vi "CRYMake Play and Record Array.vi"(0 "Play&Record/Record":bool, 1 "Name Mode":bool, 2 "Selected Record Signal Path In":string[](array[string]), 3 "Selected Play Signal Path In":string[](array[string]), 5 "Selected Record In":string[][](array[string]), 7 "input channel Info In":T5[](array[typedef]) {"Coupling" items=["Default"=-1, "RSE"=10083, "NRSE"=10078, "Differential"=10106, "Pseudodifferential"=12529]; "term config" items=["Default"=-1, "RSE"=10083, "NRSE"=10078, "Differential"=10106, "Pseudodifferential"=12529]; "Anti-aliasing Factor (%fs)" format="%.2f"}, 9 "Selected Play In":string[][](array[string]), 11 "output channel Info In":T5[](array[typedef]) {"Coupling" items=["Default"=-1, "RSE"=10083, "NRSE"=10078, "Differential"=10106, "Pseudodifferential"=12529]; "term config" items=["Default"=-1, "RSE"=10083, "NRSE"=10078, "Differential"=10106, "Pseudodifferential"=12529]; "Anti-aliasing Factor (%fs)" format="%.2f"}, 12 "Rec Time":dbl=8.0, 13 "Rec Padding Time":dbl) -> (4 "Record Cluster Out":T1, 6 "Play Cluster Out":T2, 8 "Real Rec Len":i32[](array[numeric]), 15 "Record Name Array":string[][](array[string]))   [LabVIEW 2013]
uses:
  Typedef Control/CRYHardware Channel Info.ctl
panel:
  out "size(s)":i32
  out "Sel Ch Name":string
  in  "Vp Out":dbl=2.6 min=0.1 step=0.01 format="%.2f"
  in  "Record cluster":T3={"RecDeviceID"=1, "RecSampleFreq"=2, "RecChannels"=3, "RecBitDepth"=16, "RecSampleData"=[5, 6], "RecDataLength"=6, "RecTime"=5.5, "RecLatency"=6.6, "RecPadding"=7.7, "nBufferUse"=8, "nRealTime"=9, "Anti Alias"=0, "Device Name"="", "Audio Driver"=0}
  in  "Play cluster":T4={"InSampleFreq"=44100, "nInBitDepth"=1, "nInChannels"=2, "InSignalData"=[-128.0, -127.0], "InSampleLen"=1000, "PlayDeviceID"=3, "PlaySampleFreq"=4, "PlayChannels"=5, "PlayBitDepth"=6, "PlayMode"=7, "PlayDuration"=8.0, "PlaynTimes"=9, "PlayOutLevel"=10.0, "Device Name"=""}
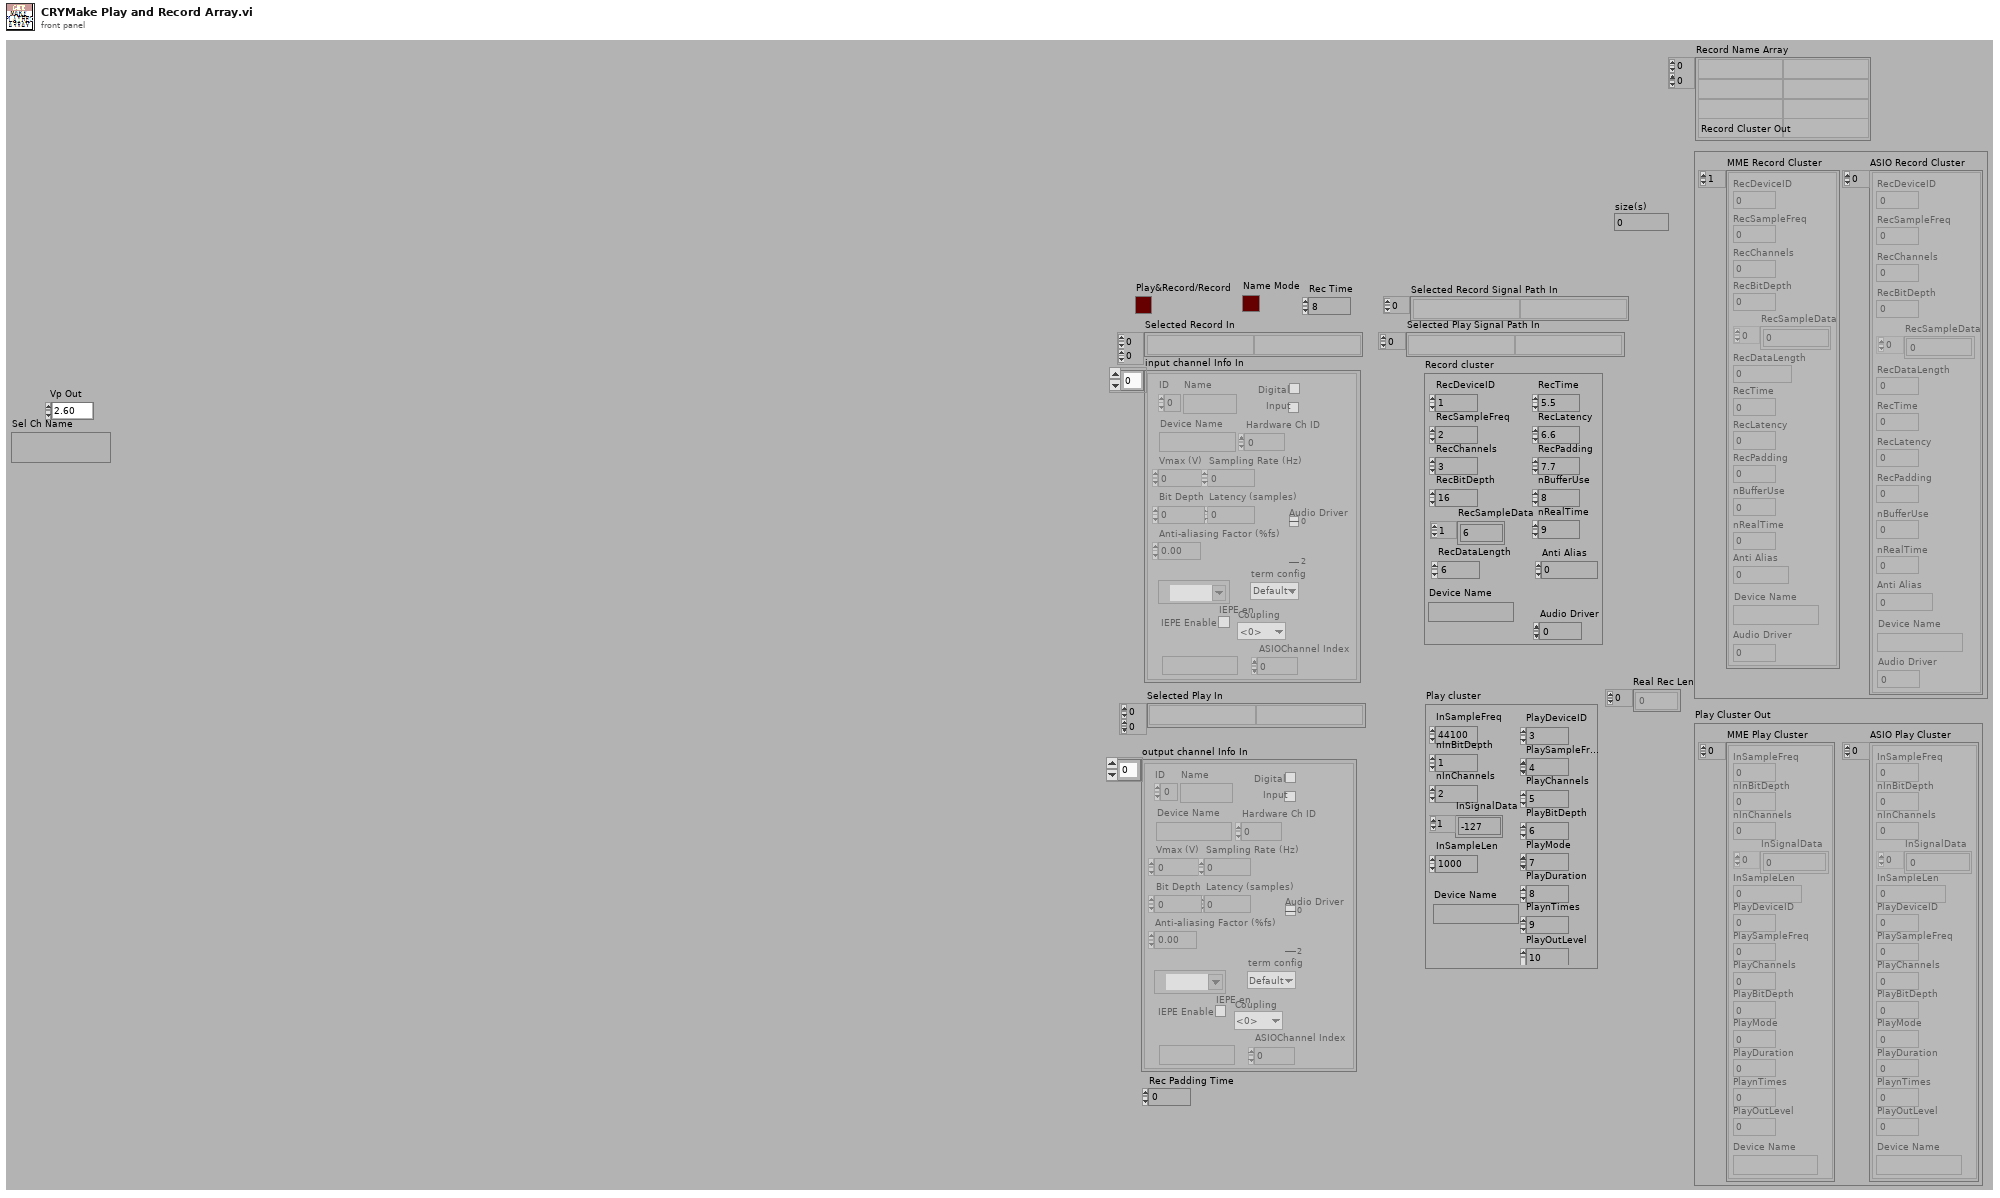
[diagram p1: front panel]
types:
  T1 = cluster{"MME Record Cluster":cluster{"RecDeviceID":u32, "RecSampleFreq":u32, "RecChannels":u32, "RecBitDepth":u32, "RecSampleData":i32[], "RecDataLength":u32, "RecTime":sgl, "RecLatency":sgl, "RecPadding":sgl, "nBufferUse":u32, "nRealTime":u32, "Anti Alias":u32, "Device Name":string, "Audio Driver":u16}[], "ASIO Record Cluster":cluster{"RecDeviceID":u32, "RecSampleFreq":u32, "RecChannels":u32, "RecBitDepth":u32, "RecSampleData":i32[], "RecDataLength":u32, "RecTime":sgl, "RecLatency":sgl, "RecPadding":sgl, "nBufferUse":u32, "nRealTime":u32, "Anti Alias":u32, "Device Name":string, "Audio Driver":u16}[]}
  T2 = cluster{"MME Play Cluster":cluster{"InSampleFreq":u32, "nInBitDepth":u32, "nInChannels":u32, "InSignalData":sgl[], "InSampleLen":u32, "PlayDeviceID":u32, "PlaySampleFreq":u32, "PlayChannels":u32, "PlayBitDepth":u32, "PlayMode":u32, "PlayDuration":sgl, "PlaynTimes":u32, "PlayOutLevel":sgl, "Device Name":string}[], "ASIO Play Cluster":cluster{"InSampleFreq":u32, "nInBitDepth":u32, "nInChannels":u32, "InSignalData":sgl[], "InSampleLen":u32, "PlayDeviceID":u32, "PlaySampleFreq":u32, "PlayChannels":u32, "PlayBitDepth":u32, "PlayMode":u32, "PlayDuration":sgl, "PlaynTimes":u32, "PlayOutLevel":sgl, "Device Name":string}[]}
  T3 = cluster{"RecDeviceID":u32, "RecSampleFreq":u32, "RecChannels":u32, "RecBitDepth":u32, "RecSampleData":i32[], "RecDataLength":u32, "RecTime":sgl, "RecLatency":sgl, "RecPadding":sgl, "nBufferUse":u32, "nRealTime":u32, "Anti Alias":u32, "Device Name":string, "Audio Driver":u16}
  T4 = cluster{"InSampleFreq":u32, "nInBitDepth":u32, "nInChannels":u32, "InSignalData":sgl[], "InSampleLen":u32, "PlayDeviceID":u32, "PlaySampleFreq":u32, "PlayChannels":u32, "PlayBitDepth":u32, "PlayMode":u32, "PlayDuration":sgl, "PlaynTimes":u32, "PlayOutLevel":sgl, "Device Name":string}
  T5 = typedef "CRYHardware Channel Info.ctl" = cluster{"ID":i32, "Name":string, "Digital":bool, "Input":bool, "Device Name":string, "Hardware Ch ID":u8, "Vmax (V)":dbl, "Latency (samples)":dbl, "Sampling Rate (Hz)":u32, "Bit Depth":u32, "Anti-aliasing Factor (%fs)":sgl, "DAQmx Channel":tag, "term config":i32, "Coupling":i32, "IEPE en":bool, "ASIOChannel Name":string, "Audio Driver":u16, "ASIOChannel Index":u8}
  T6 = cluster{"MME Record Cluster":cluster{"RecDeviceID":u32, "RecSampleFreq":u32, "RecChannels":u32, "RecBitDepth":u32, "RecSampleData":i32[], "RecDataLength":u32, "RecTime":sgl, "RecLatency":sgl, "RecPadding":sgl, "nBufferUse":u32, "nRealTime":u32, "Anti Alias":u32, "Device Name":string, "Anti Alias 2":u16}[], "ASIO Record Cluster":cluster{"RecDeviceID":u32, "RecSampleFreq":u32, "RecChannels":u32, "RecBitDepth":u32, "RecSampleData":i32[], "RecDataLength":u32, "RecTime":sgl, "RecLatency":sgl, "RecPadding":sgl, "nBufferUse":u32, "nRealTime":u32, "Anti Alias":u32, "Device Name":string, "Anti Alias 2":u16}[]}
  T7 = cluster{"RecDeviceID":u32, "RecSampleFreq":u32, "RecChannels":u32, "RecBitDepth":u32, "RecSampleData":i32[], "RecDataLength":u32, "RecTime":sgl, "RecLatency":sgl, "RecPadding":sgl, "nBufferUse":u32, "nRealTime":u32, "nRealTime 2":u32, string, "nRealTime 3":u16}[]
  T8 = cluster{"InSampleFreq":u32, "nInBitDepth":u32, "nInChannels":u32, "InSignalData":sgl[], "InSampleLen":u32, "PlayDeviceID":u32, "PlaySampleFreq":u32, "PlayChannels":u32, "PlayBitDepth":u32, "PlayMode":u32, "PlayDuration":sgl, "PlaynTimes":u32, "PlayOutLevel":sgl, string}[]
  T9 = typedef "CRYWaveform Cluster.ctl" = cluster{"Waveform":cluster{"X0":dbl, "dX":dbl, "Y":sgl[]}, "X data":u16, "Y data":u16, "Y axis":u16, "X unit":string, "Y unit":string, "Y dB ref":dbl, "display Y":bool, "display X":bool, "Overload?":bool, "Test Info":string, "Step No.":i32, "Name":string, "protected":bool, "Sqc history":string[], "Signal Channel ID":i32, "Plot Settings":cluster{"Color":u32, "Interpolation":u8, "Point Style":u8, "Line Style":u8, "Point Color":u32, "Line Width":u8, "Bar Plot Style":u8, "Fill To":i16}, "AutoProtect":bool}
  T10 = typedef "CRYCalibration 2DCluster.ctl" = cluster{"Calibration":T11, "Corr Curve":T12, "EQ Curve":T12, "Sens Curve":T12}
  T11 = typedef "CRYCalibration Cluster.ctl" = cluster{"Calibration Step Name":string, "Device":string, "Correction Curve Name":string, "Equalization Curve Name":string, "Sensitivity Curve Name":string, "Corr Folder and File":string, "EQ Folder and File":string, "Sens Folder and File":string, "Corr Step size":u16, "EQ Step size":u16, "Input":bool, "Last Cal Date (sec)":timestamp, "Cha Name":string, "Corr Curve Found":bool, "EQ Curve Found":bool, "Sens Curve Found":bool, "Signal Type":string, "Calibrated Device":string, "Hz":u32}
  T12 = typedef "CRYData Cluster.ctl" = cluster{"Name":string, "Curve":cluster{"x":dbl, "y":dbl, "z":dbl}[], "X data":u16, "Y data":u16, "Z data":u16, "X axis":u16, "Y axis":u16, "Z axis":u16, "X unit":string, "Y unit":string, "Z unit":string, "X dB ref":dbl, "Y dB ref":dbl, "Z dB ref":dbl, "single val":bool, "protected":bool, "display X":bool, "display Y":bool, "display Z":bool, "Test Info":string, "Step No.":i32, "Plot Settings":cluster{"Color":u32, "Interpolation":u8, "Point Style":u8, "Line Style":u8, "Point Color":u32, "Line Width":u8, "Bar Plot Style":u8, "Fill To":i16}, "AutoProtect":bool}
  T13 = cluster{"InSampleFreq":u32, "nInBitDepth":u32, "nInChannels":u32, "InSignalData":sgl[], "InSampleLen":u32, "PlayDeviceID":u32, "PlaySampleFreq":u32, "PlayChannels":u32, "PlayBitDepth":u32, "PlayMode":u32, "PlayDuration":sgl, "PlaynTimes":u32, "PlayOutLevel":sgl, string}
  T14 = cluster{"Sample Frequency":dbl, "Channels":i32, "bit per sample":i32}
  T15 = cluster{"RecDeviceID":u32, "RecSampleFreq":u32, "RecChannels":u32, "RecBitDepth":u32, "RecSampleData":i32[], "RecDataLength":u32, "RecTime":sgl, "RecLatency":sgl, "RecPadding":sgl, "nBufferUse":u32, "nRealTime":u32, "nRealTime 2":u32, string, "nRealTime 3":u16}
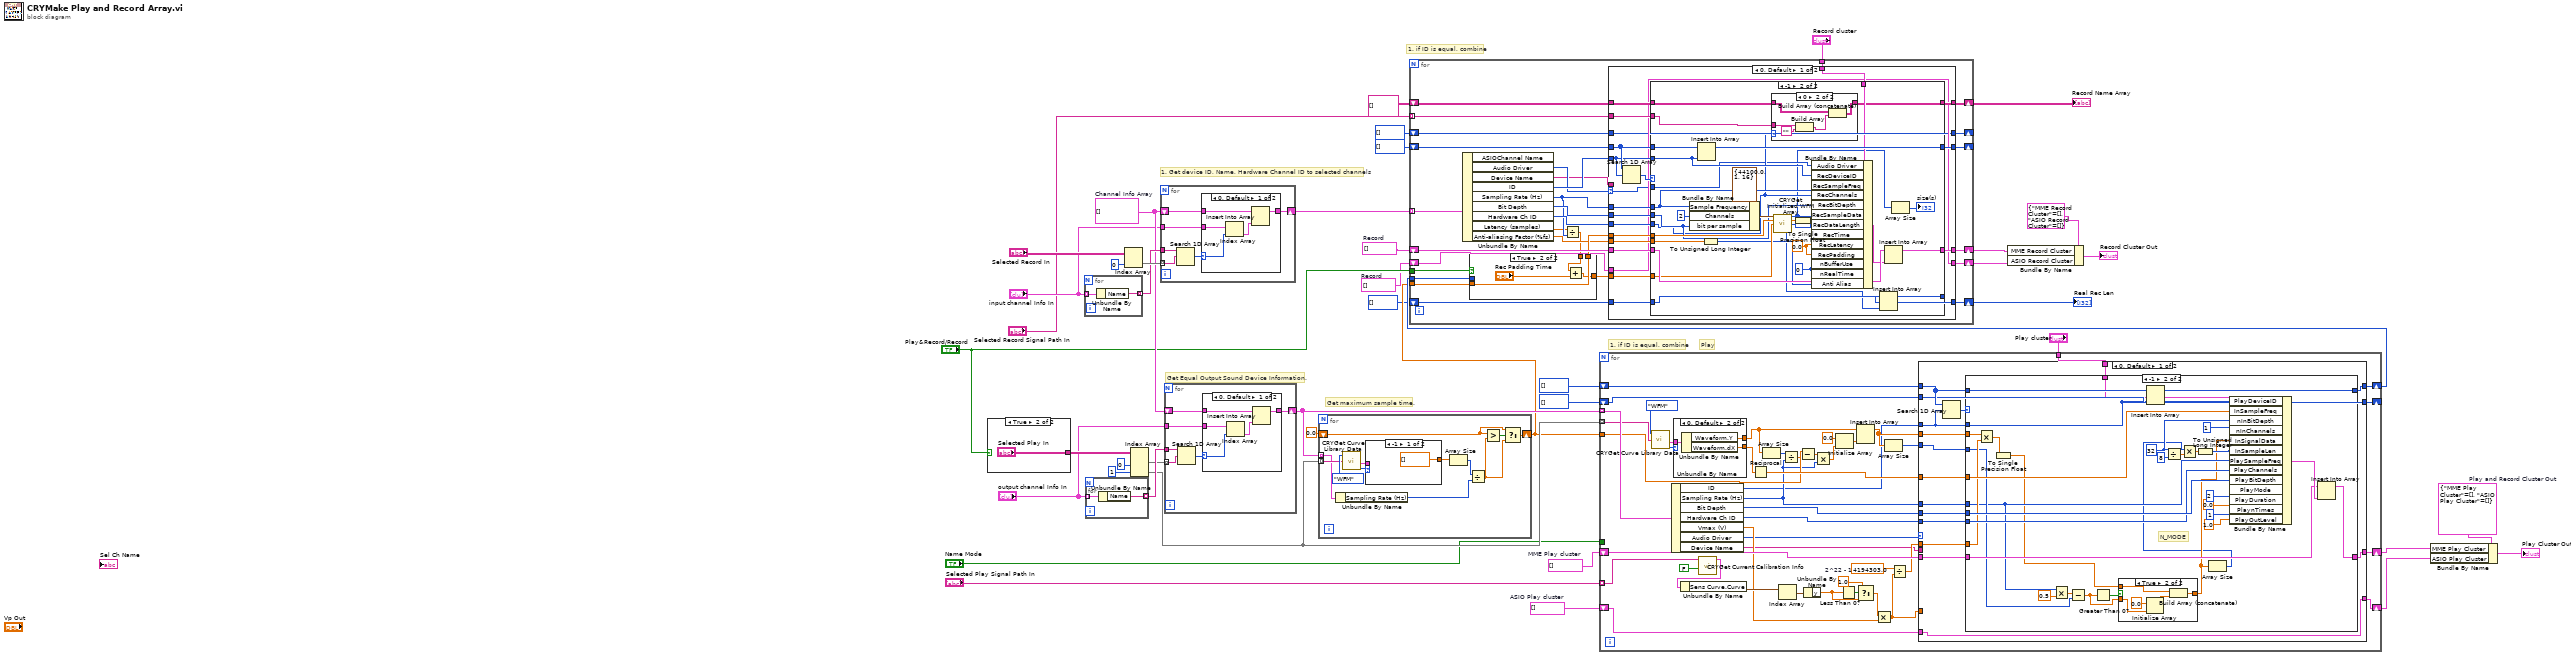
[diagram p0: block diagram]
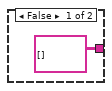
[diagram p2: hidden frame]
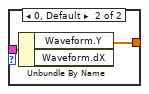
[diagram p3: hidden frame]
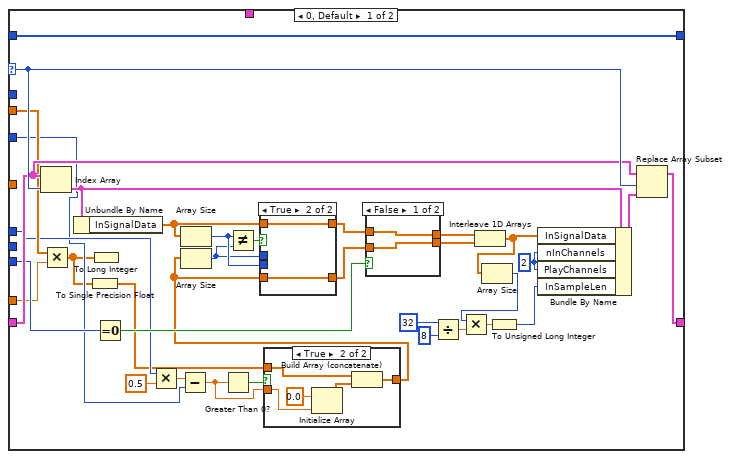
[diagram p4: hidden frame]
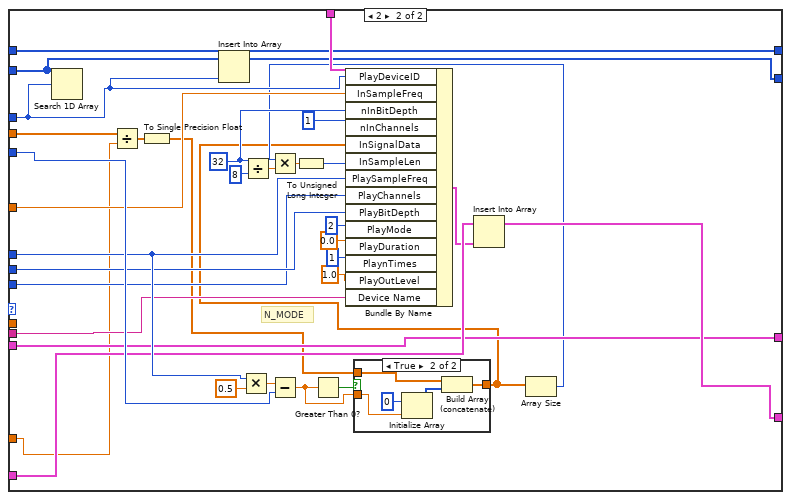
[diagram p9: hidden frame]
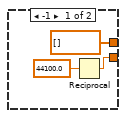
[diagram p11: hidden frame]
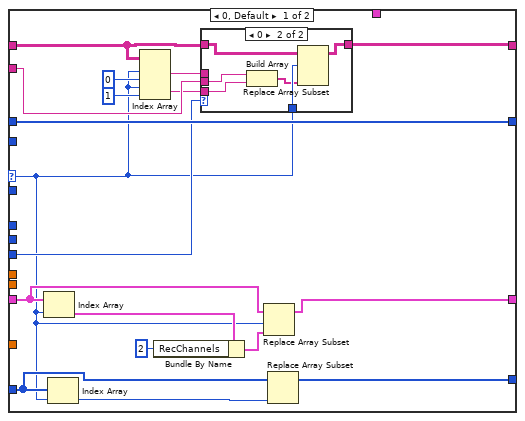
[diagram p12: hidden frame]
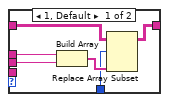
[diagram p13: hidden frame]
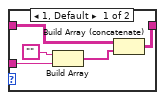
[diagram p14: hidden frame]
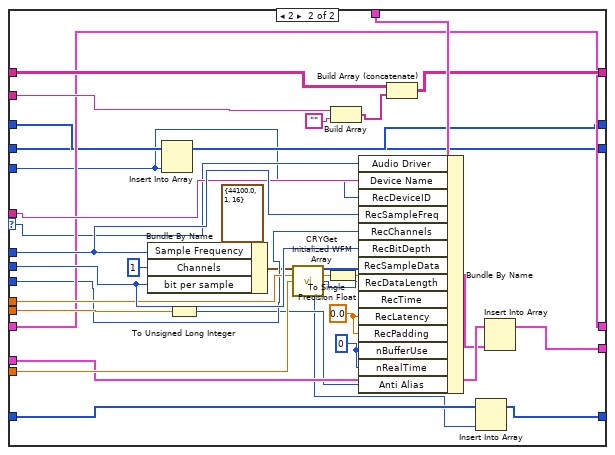
[diagram p15: hidden frame]
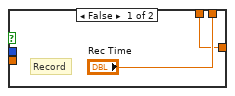
[diagram p16: hidden frame]
diagram:
  w2 = T2 {"MME Play Cluster"=[], "ASIO Play Cluster"=[]}  # Play and Record Cluster Out
  w8 = T7 []  # Record
  w11 = T8 []  # ASIO Play cluster
  w28 = T8 []  # MME Play cluster
  w29 = T7 []  # Record
  w38 = T5[] []  # Channel Info Array
  # "Play"
  # "Get maximum sample time."
  # "Get Equal Output Sound Device Information."
  # "1. if ID is equal, combine"
  # "1. if ID is equal, combine"
  # "1. Get device ID, Name, Hardware Channel ID to selected channels"
  n1 = case shown="True" "Play&Record/Record" {
    tunnel: [string[][] [] ("Selected Play In") "Selected Play In"] -> w21
    frame False {
    }
    frame True {
    }
  }
  n2 = for {
    tunnel: "input channel Info In" -> [w48] mode=indexing
    tunnel: [w47] -> w40 mode=indexing
    n3 = Unbundle By Name(w48) -> ("Name"=w47:string)
  }
  n4 = for {
    tunnel: "output channel Info In" -> [w50] mode=indexing
    tunnel: [w49] -> w44 mode=indexing
    n5 = Unbundle By Name(w50) -> ("Name"=w49:string)
  }
  n6 = Index Array(array="Selected Record In", index (col)=0 ("index")) -> (element=w41:string[])  [unwired: 1 in]
  n7 = Index Array(array=w21, index (col) #1=0 ("index"), index (col) #2=1 ("index (col)")) -> (element #1=w43:string[], element #2=w25:string[])  [unwired: 2 in]
  n8 = for {
    tunnel: w41 -> [w54] mode=indexing
    tunnel: w40 -> [w56]
    tunnel: "input channel Info In" -> [w55]
    shift-right: [w52] -> w35
    shift-left: w38 -> [w51]
    n9 = Search 1D Array(1D array=w56, element=w54) -> (index of element=w53:i32)  [unwired: 1 out]
    n10 = case shown="0, Default" w53 {
      selector: w53 -> [w60 _]
      tunnel: w55 -> [w61 _]
      tunnel: [w58 w62] -> w52
      tunnel: w51 -> [w57 w62]
      frame 0, Default {
        n11 = Index Array(array=w61, index=w60) -> (element=w59:T5)
        n12 = Insert Into Array(array=w57, new element=w59) -> (w58:T5[])  [unwired: 1 in]
      }
      frame -1 {
      }
    }
  }
  n13 = for {
    tunnel: w43 -> [w66] mode=indexing
    tunnel: w44 -> [w68]
    tunnel: "output channel Info In" -> [w67]
    shift-right: [w64] -> w26
    shift-left: w38 -> [w63]
    n14 = Search 1D Array(1D array=w68, element=w66) -> (index of element=w65:i32)  [unwired: 1 out]
    n15 = case shown="0, Default" w65 {
      selector: w65 -> [w72 _]
      tunnel: w67 -> [w73 _]
      tunnel: [w70 w74] -> w64
      tunnel: w63 -> [w69 w74]
      frame 0, Default {
        n16 = Index Array(array=w73, index=w72) -> (element=w71:T5)
        n17 = Insert Into Array(array=w69, new element=w71) -> (w70:T5[])  [unwired: 1 in]
      }
      frame -1 {
      }
    }
  }
  n18 = for {
    tunnel: w26 -> [w83] mode=indexing
    tunnel: w25 -> [w84] mode=indexing
    shift-right: [w79] -> w23
    shift-left: 0.0 -> [w78]
    n19 = Unbundle By Name(w83) -> ("Sampling Rate (Hz)"=w75:u32)
    n20 = call "CRYGet Curve Library Data.vi"("Type"=enum16{"Curves", "Values", "Results", "WFM"}."WFM", "Data Name"=w84) -> ("Wave"=w85:T9, "index"=w76:i32)  [unwired: 3 out]
    n21 = case shown="-1" w76 {
      tunnel: w85 -> [_ w89]
      tunnel: [sgl[] [] ("Y") w88] -> w82
      frame -1 {
      }
      frame 0, Default {
        n22 = Unbundle By Name(w89) -> ("Waveform.Y"=w88:sgl[])  [unwired: 1 out]
      }
    }
    n23 = Array Size(array=w82) -> (size(s)=w81:i32)
    n24 = Divide(x=w81, y=w75) -> (x/y=w77:dbl)
    n25 = Greater?(x=w78, y=w77) -> (0:w80:bool)
    n26 = Select(t=w78, s=w80, f=w77) -> (s? t:f=w79:dbl)
  }
  n27 = for {
    tunnel: w26 -> [w134] mode=indexing
    shift-right: [w132] -> w32
    shift-left: i32[] [] -> [w133]
    tunnel: w25 -> [w130] mode=indexing
    tunnel: "Play cluster" -> [w128]
    shift-right: [w91] -> w10
    shift-left: w28 -> [w127]
    tunnel: w23 -> [w111]
    tunnel: "Name Mode" -> [_]
    tunnel: "Selected Play Signal Path In" -> [w99] mode=indexing
    shift-right: [w94] -> _
    shift-left: i32[] [] -> [w97]
    shift-right: [w92] -> w9
    shift-left: w11 -> [w95]
    w100 = 4194303.0  # 2^22 - 1
    n28 = call "CRYGet Curve Library Data.vi"("Type"=enum16{"Curves", "Values", "Results", "WFM"}."WFM", "Data Name"=w130) -> ("Wave"=w131:T9, "index"=w123:i32)  [unwired: 3 out]
    n29 = Unbundle By Name(w134) -> ("ID"=w98:i32, "Sampling Rate (Hz)"=w108:u32, "Bit Depth"=w101:u32, "Hardware Ch ID"=w129:u8, "Vmax (V)"=w113:dbl, "Audio Driver"=w96:u16, "Device Name"=w93:string)
    n30 = case shown="0, Default" w123 {
      tunnel: w131 -> [_ w284]
      tunnel: [sgl[] [] ("Y") w283] -> w105
      tunnel: [w280 w282] -> w125
      frame -1 {
        n31 = Reciprocal(x=44100.0) -> (1/x=w280:dbl)
      }
      frame 0, Default {
        n32 = Unbundle By Name(w284) -> ("Waveform.Y"=w283:sgl[], "Waveform.dX"=w282:dbl)
      }
    }
    n33 = call "CRYGet Current Calibration Info.vi"("Is Input?"=FALSE, "Signal Type Name"=w99) -> ("Calibration All Cluster"=w118:T10)  [unwired: 9 out]
    n34 = Unbundle By Name(w118) -> ("Sens Curve.Curve"=w121:cluster{"x":dbl, "y":dbl, "z":dbl}[])
    n35 = Reciprocal(x=w125) -> (1/x=w124:dbl)
    n36 = Array Size(array=w105) -> (size(s)=w112:i32)
    n37 = Index Array(array=w121) -> (element=w120:cluster{"x":dbl, "y":dbl, "z":dbl})  [unwired: 1 in]
    n38 = Divide(x=w112, y=w108) -> (x/y=w110:dbl)
    n39 = Subtract(x=w111, y=w110) -> (x-y=w109:dbl)
    n40 = Unbundle By Name(w120) -> ("y"=w115:dbl)
    n41 = Multiply(x=w109, y=w108) -> (x*y=w107:dbl)
    n42 = Initialize Array(sgl 0.0 ("element"), w107) -> (w104:sgl[])
    n43 = Less Than 0?(x=w115) -> (x < 0?=w117:bool)
    n44 = Insert Into Array(array=w105, new element=w104) -> (w103:sgl[])  [unwired: 1 in]
    n45 = Select(t=1.0, s=w117, f=w115) -> (s? t:f=w114:dbl)
    n46 = Multiply(x=w114, y=w113) -> (x*y=w90:dbl)
    n47 = Array Size(array=w103) -> (size(s)=w126:i32)
    n48 = Divide(x=w100, y=w90) -> (x/y=w102:dbl)
    n49 = case shown="0, Default" w96 {
      tunnel: w133 -> [w150 w263]
      tunnel: [w148 w263] -> w132
      tunnel: w129 -> [w147 w259]
      tunnel: w128 -> [w146 w272]
      tunnel: [w135 w271] -> w92
      tunnel: w127 -> [w145 w260]
      tunnel: w126 -> [w144 w270]
      tunnel: w124 -> [w143 w269]
      tunnel: w108 -> [w142 w268]
      tunnel: w103 -> [w141 w267]
      tunnel: w102 -> [w140 _]
      tunnel: w101 -> [w139 w266]
      tunnel: w98 -> [w138 w258]
      tunnel: w97 -> [w137 w265]
      tunnel: w95 -> [w135 w261]
      tunnel: [w137 w264] -> w94
      tunnel: w93 -> [_ w262]
      tunnel: [w136 w260] -> w91
      tunnel: w90 -> [_ w238]
      frame 0, Default {
        n50 = Search 1D Array(1D array=w150, element=w138) -> (index of element=w149:i32)  [unwired: 1 out]
        n51 = case shown="-1" w149 {
          selector: w149 -> [w182 _]
          tunnel: w150 -> [w185 w231]
          tunnel: [w185 w230] -> w148
          tunnel: w138 -> [_ w210]
          tunnel: w147 -> [w174 w215]
          tunnel: w139 -> [_ w217]
          tunnel: w146 -> [_ w220]
          tunnel: [w180 w214] -> w136
          tunnel: w145 -> [w181 w218]
          tunnel: w142 -> [w155 w205]
          tunnel: w144 -> [w154 w206]
          tunnel: w141 -> [w161 w213]
          tunnel: w143 -> [_ w216]
          tunnel: w140 -> [w160 w211]
          frame 0, Default {
            w173 = u32 2 ("PlayChannels")
            n52 = Index Array(array=w181, index=w182) -> (element=w184:T13)
            n53 = Multiply(x=w161, y=w160) -> (x*y=w152:dbl[])
            n54 = Unbundle By Name(w184) -> ("InSignalData"=w177:sgl[])
            n55 = To Single Precision Float(number=w152) -> (single precision float=w151:sgl[])
            n56 = To Long Integer(number=w152) -> ()  [unwired: 1 out]
            n57 = Equal To 0?(x=w174) -> (x = 0?=w179:bool)
            n58 = Multiply(x=w155, y=0.5) -> (x*y=w158:dbl)
            n59 = Subtract(x=w158, y=w154) -> (x-y=w159:dbl)
            n60 = Array Size(array=w177) -> (size(s)=w176:i32)
            n61 = Greater Than 0?(x=w159) -> (x > 0?=w156:bool)
            n62 = case shown="True" w156 {
              tunnel: w151 -> [w186 w187]
              tunnel: w159 -> [_ w191]
              tunnel: [w186 w188] -> w153
              frame False {
              }
              frame True {
                n63 = Initialize Array(sgl 0.0, w191) -> (w189:sgl[])
                n64 = Build Array (concatenate)(w187, w189) -> (w188:sgl[])
              }
            }
            n65 = Array Size(array=w153) -> (size(s)=w175:i32)
            n66 = Not Equal?(x=w176, y=w175) -> (x != y?=w178:bool)
            n67 = case shown="True" w178 {
              tunnel: w176 -> [_ _]
              tunnel: w153 -> [w193 w194]
              tunnel: [w193 w194] -> w163
              tunnel: w177 -> [w192 w195]
              tunnel: [w192 w195] -> w162
              tunnel: w175 -> [_ _]
              frame False {
              }
              frame True {
              }
            }
            n68 = case shown="False" w179 {
              tunnel: w162 -> [w197 w199]
              tunnel: w163 -> [w196 w198]
              tunnel: [w196 w199] -> w171
              tunnel: [w197 w198] -> w172
              frame False {
              }
              frame True {
              }
            }
            n69 = Divide(x=u32 32, y=u32 8) -> (x/y=w168:dbl)
            n70 = Interleave 1D Arrays(w172, w171) -> (w170:sgl[])
            n71 = Array Size(array=w170) -> (size(s)=w166:i32)
            n72 = Multiply(x=w166, y=w168) -> (x*y=w169:dbl)
            n73 = To Unsigned Long Integer(number=w169) -> (unsigned 32bit integer=w164:u32)
            n74 = Bundle By Name(cluster=w184, "InSignalData"=w170, "nInChannels"=w173, "PlayChannels"=w173, "InSampleLen"=w164) -> (w183:T13)
            n75 = Replace Array Subset(array=w181, new element=w183, index=w182) -> (w180:T8)
          }
          frame -1 {
            w223 = u32 32 ("x")
            # "N_MODE"
            n76 = Multiply(x=w213, y=w211) -> (x*y=w201:dbl[])
            n77 = To Single Precision Float(number=w201) -> (single precision float=w200:sgl[])
            n78 = Multiply(x=w205, y=0.5) -> (x*y=w208:dbl)
            n79 = Subtract(x=w208, y=w206) -> (x-y=w209:dbl)
            n80 = Greater Than 0?(x=w209) -> (x > 0?=w204:bool)
            n81 = case shown="True" w204 {
              tunnel: w200 -> [w232 w233]
              tunnel: w209 -> [_ w237]
              tunnel: [w232 w234] -> w203
              frame False {
              }
              frame True {
                n82 = Initialize Array(sgl 0.0, w237) -> (w235:sgl[])
                n83 = Build Array (concatenate)(w233, w235) -> (w234:sgl[])
              }
            }
            n84 = Insert Into Array(array=w231, new element=w210) -> (w230:i32[])  [unwired: 1 in]
            n85 = Divide(x=w223, y=u32 8) -> (x/y=w224:dbl)
            n86 = Array Size(array=w203) -> (size(s)=w202:i32)
            n87 = Multiply(x=w202, y=w224) -> (x*y=w225:dbl)
            n88 = To Unsigned Long Integer(number=w225) -> (unsigned 32bit integer=w222:u32)
            n89 = Bundle By Name(cluster=w220, "PlayDeviceID"=w210, "InSampleFreq"=w216, "nInBitDepth"=w223, "nInChannels"=u32 1, "InSignalData"=w203, "InSampleLen"=w222, "PlaySampleFreq"=w205, "PlayChannels"=w215, "PlayBitDepth"=w217, "PlayMode"=u32 2, "PlayDuration"=sgl 0.0, "PlaynTimes"=u32 1, "PlayOutLevel"=sgl 1.0) -> (w219:T4)
            n90 = Insert Into Array(array=w218, new element=w219) -> (w214:T8)  [unwired: 1 in]
          }
        }
      }
      frame 2 {
        w251 = u32 32 ("x")
        # "N_MODE"
        n91 = Search 1D Array(1D array=w265, element=w258) -> ()  [unwired: 2 out]
        n92 = Divide(x=w267, y=w238) -> (x/y=w246:dbl[])
        n93 = To Single Precision Float(number=w246) -> (single precision float=w242:sgl[])
        n94 = Insert Into Array(array=w265, new element=w258) -> (w264:i32[])  [unwired: 1 in]
        n95 = Multiply(x=w268, y=0.5) -> (x*y=w244:dbl)
        n96 = Divide(x=w251, y=u32 8) -> (x/y=w252:dbl)
        n97 = Subtract(x=w244, y=w270) -> (x-y=w245:dbl)
        n98 = Greater Than 0?(x=w245) -> (x > 0?=w241:bool)
        n99 = case shown="True" w241 {
          tunnel: w242 -> [w273 w274]
          tunnel: w245 -> [_ w278]
          tunnel: [w273 w275] -> w239
          frame False {
          }
          frame True {
            n100 = Initialize Array(0, w278) -> (w276:i32[])
            n101 = Build Array (concatenate)(w274, w276) -> (w275:sgl[])
          }
        }
        n102 = Array Size(array=w239) -> (size(s)=w240:i32)
        n103 = Multiply(x=w240, y=w252) -> (x*y=w253:dbl)
        n104 = To Unsigned Long Integer(number=w253) -> (unsigned 32bit integer=w250:u32)
        n105 = Bundle By Name(cluster=w272, "PlayDeviceID"=w258, "InSampleFreq"=w269, "nInBitDepth"=w251, "nInChannels"=u32 1, "InSignalData"=w239, "InSampleLen"=w250, "PlaySampleFreq"=w268, "PlayChannels"=w259, "PlayBitDepth"=w266, "PlayMode"=u32 2, "PlayDuration"=sgl 0.0, "PlaynTimes"=u32 1, "PlayOutLevel"=sgl 1.0, "Device Name"=w262) -> (w248:T4)
        n106 = Insert Into Array(array=w261, new element=w248) -> (w271:T8)  [unwired: 1 in]
      }
    }
  }
  n107 = for {
    tunnel: w35 -> [w313] mode=indexing
    shift-right: [w312] -> _
    shift-left: i32[] [] -> [w311]
    shift-right: [w291] -> w5
    shift-left: w29 -> [w310]
    tunnel: "Record cluster" -> [w308]
    tunnel: w32 -> [w306]
    tunnel: "Play&Record/Record" -> [w303]
    tunnel: w23 -> [w302]
    shift-right: [w299] -> w18
    shift-left: i32[] [] -> [w298]
    tunnel: "Selected Record Signal Path In" -> [w297] mode=indexing
    shift-right: [w295] -> w14
    shift-left: string[][] [] ("Array") -> [w296]
    shift-right: [w290] -> w6
    shift-left: w8 -> [w292]
    shift-right: [w288] -> _
    shift-left: i32[] [] -> [w289]
    n108 = Unbundle By Name(w313) -> ("Audio Driver"=w294:u16, "Device Name"=w293:string, "ID"=w305:i32, "Sampling Rate (Hz)"=w287:u32, "Bit Depth"=w309:u32, "Hardware Ch ID"=w307:u8, "Latency (samples)"=w286:dbl, "Anti-aliasing Factor (%fs)"=w300:sgl)  [unwired: 1 out]
    n109 = Divide(x=w286, y=w287) -> (x/y=w285:dbl)
    n110 = case shown="True" w303 {
      tunnel: w306 -> [_ _]
      tunnel: ["Rec Time" w446] -> w304
      tunnel: w302 -> [_ w446]
      tunnel: [w441 w443] -> w301
      tunnel: w285 -> [w441 w445]
      frame False {
        # "Record"
      }
      frame True {
        n111 = Add(x=w445, y="Rec Padding Time") -> (x+y=w443:dbl)
      }
    }
    n112 = case shown="0, Default" w294 {
      selector: w294 -> [w314 w422]
      tunnel: [w334 w423] -> w312
      tunnel: w311 -> [w319 w423]
      tunnel: [w333 w426] -> w291
      tunnel: w310 -> [w332 w426]
      tunnel: w287 -> [w331 w440]
      tunnel: w309 -> [w330 w439]
      tunnel: w308 -> [w329 w438]
      tunnel: w307 -> [w328 w421]
      tunnel: w305 -> [w318 w420]
      tunnel: w304 -> [w327 w437]
      tunnel: w301 -> [w326 w436]
      tunnel: w300 -> [w325 w435]
      tunnel: [w324 w434] -> w299
      tunnel: w298 -> [w323 w433]
      tunnel: w297 -> [w322 w432]
      tunnel: w296 -> [w321 w431]
      tunnel: [w320 w430] -> w295
      tunnel: w293 -> [_ w429]
      tunnel: w292 -> [w316 w428]
      tunnel: [w316 w427] -> w290
      tunnel: w289 -> [w315 w425]
      tunnel: [w315 w424] -> w288
      frame 0, Default {
        n113 = Search 1D Array(1D array=w319, element=w318) -> (index of element=w317:i32)  [unwired: 1 out]
        n114 = case shown="-1" w317 {
          selector: w317 -> [w335 _]
          tunnel: [w348 w395] -> w334
          tunnel: w319 -> [w348 w394]
          tunnel: w318 -> [_ w382]
          tunnel: [w350 w383] -> w333
          tunnel: w332 -> [w351 w385]
          tunnel: w331 -> [_ w380]
          tunnel: w330 -> [_ w378]
          tunnel: w329 -> [_ w381]
          tunnel: w328 -> [w343 w371]
          tunnel: w327 -> [_ w379]
          tunnel: w326 -> [_ w377]
          tunnel: w325 -> [_ w376]
          tunnel: [w344 w372] -> w324
          tunnel: w323 -> [w346 w374]
          tunnel: w322 -> [w338 w370]
          tunnel: w321 -> [w340 w369]
          tunnel: [w336 w368] -> w320
          tunnel: w314 -> [_ w367]
          frame 0, Default {
            n115 = Index Array(array=w351, index=w335) -> (element=w347:T15)
            n116 = Index Array(array=w346, index=w335) -> (element=w345:i32)
            n117 = Index Array(array=w340, index (row) #1=w335, index (col) #1=0 ("disabled index (col)"), index (row) #2=w335, index (col) #2=1 ("disabled index (col)")) -> (element #1=w339:string, element #2=w337:string)
            n118 = Bundle By Name(cluster=w347, "RecChannels"=u32 2) -> (w352:T15)
            n119 = case shown="0" w343 {
              tunnel: w340 -> [w355 w362]
              tunnel: [w353 w359] -> w336
              tunnel: w339 -> [w358 _]
              tunnel: w338 -> [w357 w364]
              tunnel: w337 -> [_ w363]
              tunnel: w335 -> [w354 w361]
              frame 1, Default {
                n120 = Build Array(w358, w357) -> (w356:string[])
                n121 = Replace Array Subset(array=w355, new element=w356, index (row)=w354) -> (w353:string[][])  [unwired: 1 in]
              }
              frame 0 {
                n122 = Build Array(w364, w363) -> (w360:string[])
                n123 = Replace Array Subset(array=w362, new element=w360, index (row)=w361) -> (w359:string[][])  [unwired: 1 in]
              }
            }
            n124 = Replace Array Subset(array=w351, new element=w352, index=w335) -> (w350:T7)
            n125 = Replace Array Subset(array=w346, new element=w345) -> (w344:i32[])  [unwired: 1 in]
          }
          frame -1 {
            w393 = sgl 0.0 ("RecTime")
            w392 = u32 0 ("nBufferUse")
            n126 = Bundle By Name(cluster=T14 {"Sample Frequency"=44100.0, "Channels"=1, "bit per sample"=16} ("Sound Format"), "Sample Frequency"=w380, "Channels"=2, "bit per sample"=w378) -> (w391:T14)
            n127 = Insert Into Array(array=w394, new element=w382) -> (w395:i32[])  [unwired: 1 in]
            n128 = To Unsigned Long Integer(number=w376) -> (unsigned 32bit integer=w375:u32)
            n129 = case shown="0" w371 {
              tunnel: w370 -> [w400 w405]
              tunnel: w369 -> [w398 w403]
              tunnel: [w396 w401] -> w368
              frame 1, Default {
                n130 = Build Array("" ("element"), w400) -> (w397:string[])
                n131 = Build Array (concatenate)(w398, w397) -> (w396:string[][])
              }
              frame 0 {
                n132 = Build Array(w405, "" ("element")) -> (w402:string[])
                n133 = Build Array (concatenate)(w403, w402) -> (w401:string[][])
              }
            }
            n134 = call "CRYGet Initialized WFM Array.vi"("Sound Format"=w391, "Time(s)"=w379, "Rec Padding Time"=w377) -> ("initialized array"=w366:i32[], "Time out"=w387:dbl, "Record Data Length"=w388:u32, "real size"=w373:i32)  [unwired: 9 out]
            n135 = To Single Precision Float(number=w387) -> (single precision float=w389:sgl)
            n136 = Bundle By Name(cluster=w381, "Audio Driver"=w367, "RecDeviceID"=w382, "RecSampleFreq"=w380, "RecChannels"=w371, "RecBitDepth"=w378, "RecSampleData"=w366, "RecDataLength"=w388, "RecTime"=w389, "RecLatency"=w393, "RecPadding"=w393, "nBufferUse"=w392, "nRealTime"=w392, "Anti Alias"=w375) -> (w384:T3)
            n137 = Insert Into Array(array=w374, new element=w373) -> (w372:i32[])  [unwired: 1 in]
            n138 = Insert Into Array(array=w385, new element=w384) -> (w383:T7)  [unwired: 1 in]
            n139 = Array Size(array=w366) -> (size(s)=→"size(s)":i32)
          }
        }
      }
      frame 2 {
        w419 = sgl 0.0 ("RecTime")
        w418 = u32 0 ("nBufferUse")
        n140 = Bundle By Name(cluster=T14 {"Sample Frequency"=44100.0, "Channels"=1, "bit per sample"=16} ("Sound Format"), "Sample Frequency"=w440, "Channels"=1, "bit per sample"=w439) -> (w417:T14)
        n141 = Insert Into Array(array=w425, new element=w420) -> (w424:i32[])  [unwired: 1 in]
        n142 = To Unsigned Long Integer(number=w435) -> (unsigned 32bit integer=w409:u32)
        n143 = call "CRYGet Initialized WFM Array.vi"("Sound Format"=w417, "Time(s)"=w437, "Rec Padding Time"=w436) -> ("initialized array"=w413:i32[], "Time out"=w412:dbl, "Record Data Length"=w414:u32, "real size"=w408:i32)  [unwired: 9 out]
        n144 = To Single Precision Float(number=w412) -> (single precision float=w415:sgl)
        n145 = Build Array(w432, "" ("element")) -> (w406:string[])
        n146 = Bundle By Name(cluster=w438, "Audio Driver"=w422, "Device Name"=w429, "RecDeviceID"=w420, "RecSampleFreq"=w440, "RecChannels"=w421, "RecBitDepth"=w439, "RecSampleData"=w413, "RecDataLength"=w414, "RecTime"=w415, "RecLatency"=w419, "RecPadding"=w419, "nBufferUse"=w418, "nRealTime"=w418, "Anti Alias"=w409) -> (w410:T3)
        n147 = Build Array (concatenate)(w431, w406) -> (w430:string[][])
        n148 = Insert Into Array(array=w433, new element=w408) -> (w434:i32[])  [unwired: 1 in]
        n149 = Insert Into Array(array=w428, new element=w410) -> (w427:T7)  [unwired: 1 in]
      }
    }
  }
  "Real Rec Len" <- w18
  "Record Name Array" <- w14
  n150 = Bundle By Name(cluster=T6 {"MME Record Cluster"=[], "ASIO Record Cluster"=[]} ("Record Cluster Out"), "MME Record Cluster"=w5, "ASIO Record Cluster"=w6) -> (→"Record Cluster Out":T6)
  n151 = Bundle By Name(cluster=w2, "MME Play Cluster"=w10, "ASIO Play Cluster"=w9) -> (→"Play Cluster Out":T2)
